vi "test.vi"   [LabVIEW 2012]
uses:
  <vilib>/NXT/Subs/MotorOutput.ctl
  <vilib>/NXT/Dual Mode Library/Motors/MotorOn.vi
  <vilib>/NXT/Dual Mode Library/Motors/MotorReverse.vi
  <vilib>/NXT/Dual Mode Library/Waits/Wait_Num.vi
types:
  T1 = typedef "MotorOutput.ctl" = u8
  T2 = typedef "LVHSConnector.ctl" = cluster{"Hardware":string, "Flattened String":string}
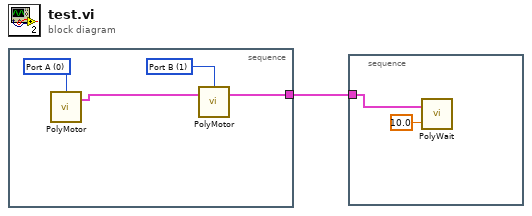
[diagram p0: block diagram]
diagram:
  n1 = stacked-sequence {
    tunnel: [w4] -> w1
    frame #0 {
      w2 = T1 1 items=["Port A"=0, "Port B"=1, "Port C"=2, "Ports A & B"=4, "Ports A & C"=5, "Ports B & C"=6, "All Ports"=3] ("Output Port (All Ports)")
      w3 = T1 0 items=["Port A"=0, "Port B"=1, "Port C"=2, "Ports A & B"=4, "Ports A & C"=5, "Ports B & C"=6, "All Ports"=3] ("Output Port (All Ports)")
      n2 = call-poly <vilib>:"PolyMotor.vi"("Output Port (All Ports)"=w3) -> ("NXT"=w5:T2)  [unwired: 3 in]
      n3 = call-poly <vilib>:"PolyMotor.vi"("NXT"=w5, "Output Port (All Ports)"=w2) -> ("NXT"=w4:T2)  [unwired: 2 in]
    }
  }
  n4 = stacked-sequence {
    tunnel: w1 -> [w7]
    frame #0 {
      n5 = call-poly <vilib>:"PolyWait.vi"("Time (1 sec)"=sgl 10.0, "NXT"=w7) -> ()  [unwired: 2 in, 1 out]
    }
  }
